vi "coincidenceVsDelay.vi"() -> ()   [LabVIEW 2020]
uses:
  <vilib>/Math Plots/2D Math Plots/2D Error Bar/2D Error Bar XCtrl/2D Error Bar.xctl
  C:/Program Files/Dotfast Consulting/Timetag Explorer 2.26/ttInterface.dll
  Program Files/Dotfast Consulting/Timetag Explorer 2.26/ttInterface.dll
  <vilib>/Utility/file.llb/Write Delimited Spreadsheet (I64).vi
  <vilib>/Math Plots/2D Math Plots/2D Error Bar/2D Error Bar Datatype/Public/Plot Helper (Fixed).vi
  <vilib>/Analysis/NI_AALBase.lvlib
  <vilib>/Math Plots/2D Math Plots/2D Error Bar/2D Error Bar Datatype/2D Error Bar Datatype.lvclass
panel:
  in  "stop":bool
  in  "Boolean":bool=TRUE
  in  "Step Delay(ns)":dbl
  in  "Stop Delay (ns)":dbl
  in  "StartDelay (ns)":dbl
  in  "fileName":string
  in  "Folder":path
  out "ChB Delay (uqd Unit)":i32
  out "ChADelay(uqd Unit)":i32
  in  "chB delay (ns)":dbl
  in  "chA delay(ns)":dbl
  in  "Ch B":u8=1 min=1 max=16 step=1
  in  "Ch A":u8=1 min=1 max=16 step=1
  out "CTW (uqd units)":i32
  in  "CTW in ns":dbl
  out "2D Error Bar":refnum<class "2D Plot Datatype.lvclass">[](xcontrol)
  out "Coincidence Rate AvsB":dbl format="%#_4p"
  out "ChB Rate":dbl format="%#_4p"
  out "ChARate":dbl format="%#_4p"
  out "Coincidence AvsB":i32
  out "Ch A":i32
  out "GetTimeCounter":i32
  out "Ch B":i32
  out "GetResolution":dbl
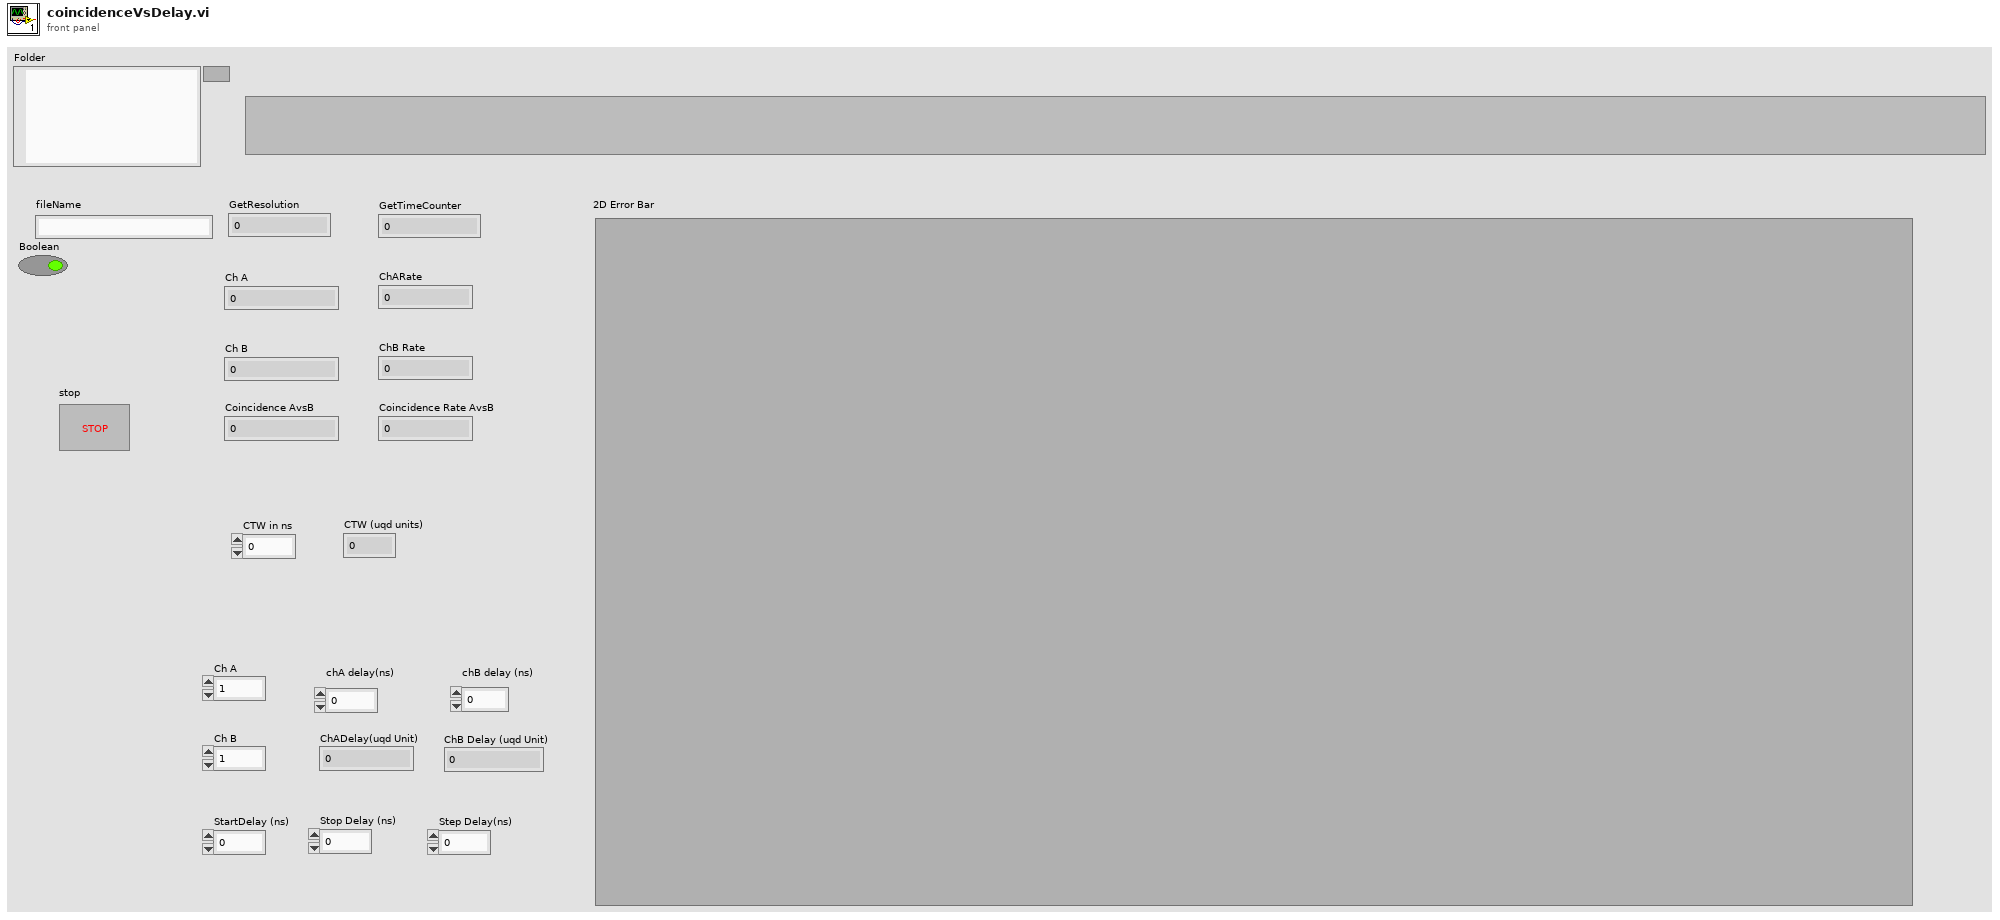
[diagram p1: front panel]
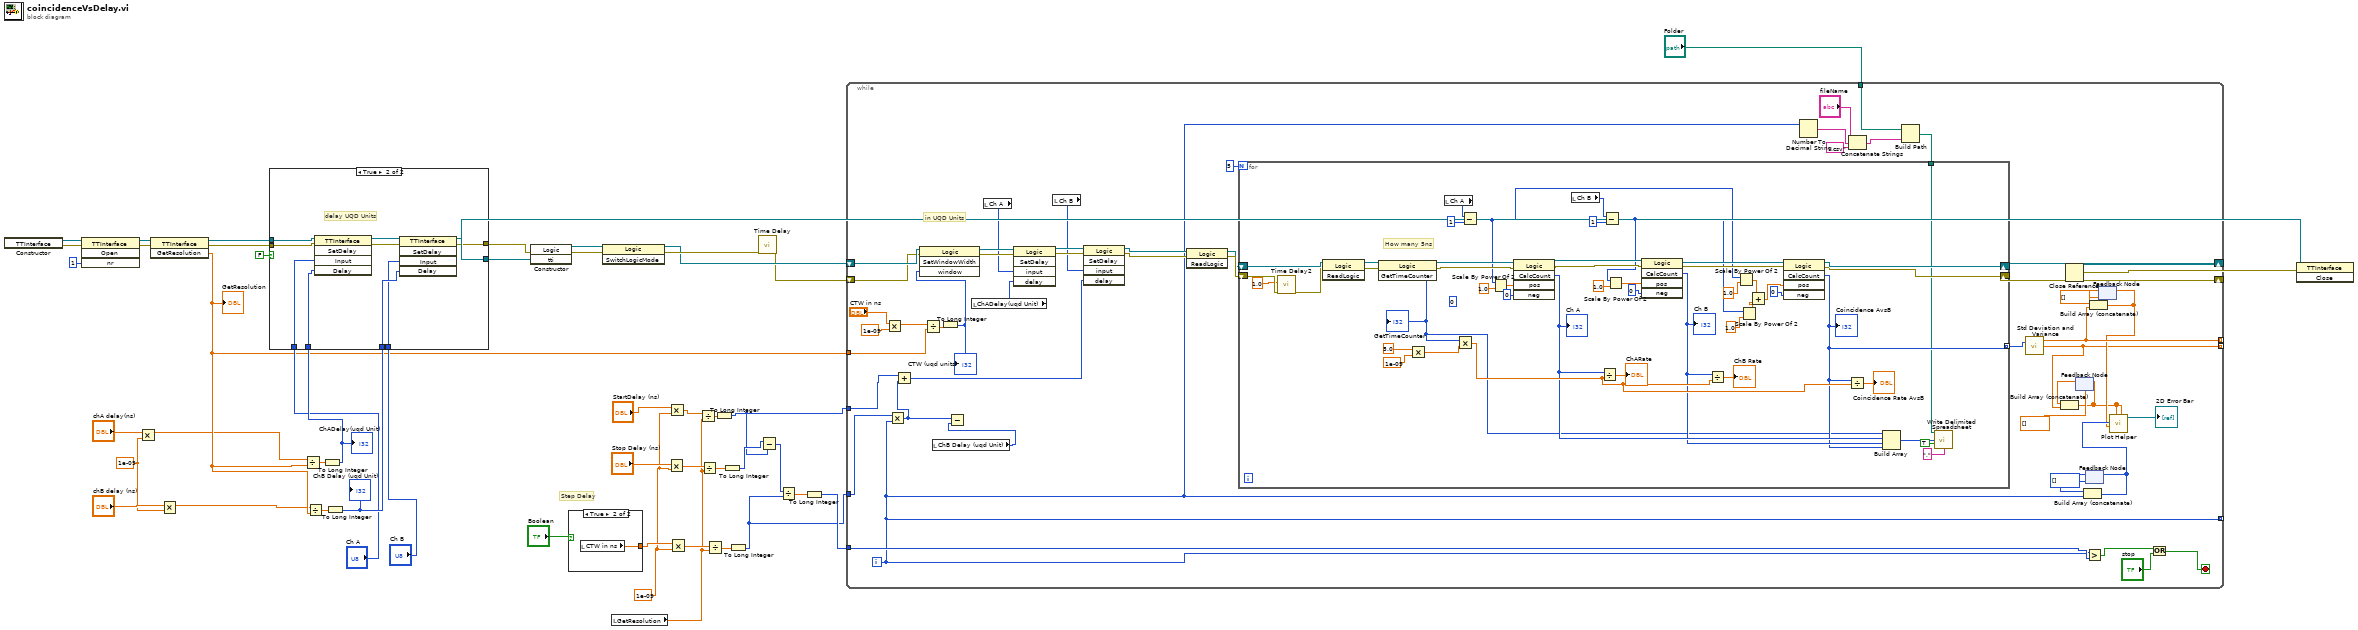
[diagram p0: block diagram]
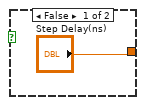
[diagram p2: hidden frame]
diagram:
  w14 = 1e-09
  w20 = 1e-09
  # "Step Delay"
  n1 = constructor class="TTInterface"() -> (reference out=w49:refnum<k24>, error out=w48:errorcluster)  [unwired: 3 in, 1 out]
  n2 = invoke class="TTInterface" method="Open"(reference=w49, error in=w48, "nr"=1) -> (reference out=w45:refnum<k24>, error out=w46:errorcluster)  [unwired: 1 in, 2 out]
  n3 = Multiply(x="chA delay(ns)", y=w20) -> (x*y=w22:dbl)
  n4 = invoke class="TTInterface" method="GetResolution"(reference=w45, error in=w46) -> (reference out=w44:refnum<k24>, error out=w43:errorcluster, "GetResolution"=w23:dbl)  [unwired: 1 in]
  "GetResolution" <- w23
  n5 = Multiply(x="chB delay (ns)", y=w20) -> (x*y=w21:dbl)
  n6 = Divide(x=w22, y=w23) -> (x/y=w29:dbl)
  n7 = Divide(x=w21, y=w23) -> (x/y=w28:dbl)
  n8 = To Long Integer(number=w29) -> (32bit integer=w27:i32)
  "ChADelay(uqd Unit)" <- w27
  n9 = To Long Integer(number=w28) -> (32bit integer=w26:i32)
  "ChB Delay (uqd Unit)" <- w26
  n10 = case shown="True" FALSE {
    tunnel: w44 -> [w51 w61]
    tunnel: w43 -> [w50 w60]
    tunnel: [w50 w57] -> w42
    tunnel: [w51 w56] -> w39
    tunnel: w27 -> [_ w55]
    tunnel: w26 -> [_ w54]
    tunnel: "Ch A" -> [_ w53]
    tunnel: "Ch B" -> [_ w52]
    frame False {
    }
    frame True {
      # "delay UQD Units"
      n11 = invoke class="TTInterface" method="SetDelay"(reference=w61, error in=w60, "Input"=w53, "Delay"=w55) -> (reference out=w59:refnum<k24>, error out=w58:errorcluster)  [unwired: 1 in, 3 out]
      n12 = invoke class="TTInterface" method="SetDelay"(reference=w59, error in=w58, "Input"=w52, "Delay"=w54) -> (reference out=w56:refnum<k24>, error out=w57:errorcluster)  [unwired: 1 in, 3 out]
    }
  }
  n13 = constructor class="Logic"(error in=w42, "tti"=w39) -> (reference out=w41:refnum<k24>, error out=w40:errorcluster)  [unwired: 2 in, 2 out]
  n14 = case shown="True" "Boolean" {
    tunnel: ["Step Delay(ns)" w63] -> w15
    frame False {
    }
    frame True {
      n15 = local read "CTW in ns"() -> (w63:dbl)
    }
  }
  n16 = invoke class="Logic" method="SwitchLogicMode"(reference=w41, error in=w40) -> (reference out=w34:refnum<k24>, error out=w35:errorcluster)  [unwired: 1 in, 1 out]
  n17 = local read "GetResolution"() -> (w10:dbl)
  n18 = Multiply(x="Stop Delay (ns)", y=w14) -> (x*y=w11:dbl)
  n19 = Multiply(x="StartDelay (ns)", y=w14) -> (x*y=w13:dbl)
  n20 = Multiply(x=w15, y=w14) -> (x*y=w12:dbl)
  n21 = Divide(x=w13, y=w10) -> (x/y=w9:dbl)
  n22 = Divide(x=w11, y=w10) -> (x/y=w8:dbl)
  n23 = Divide(x=w12, y=w10) -> (x/y=w7:dbl)
  n24 = To Long Integer(number=w9) -> (32bit integer=w3:i32)
  n25 = To Long Integer(number=w8) -> (32bit integer=w4:i32)
  n26 = To Long Integer(number=w7) -> (32bit integer=w1:i32)
  n27 = call "Time Delay"("error in (no error)"=w35) -> ("error out"=w33:errorcluster)  [unwired: 10 in]
  n28 = Subtract(x=w4, y=w3) -> (x-y=w6:i32)
  n29 = Divide(x=w6, y=w1) -> (x/y=w5:dbl)
  n30 = To Long Integer(number=w5) -> (32bit integer=w2:i32)
  n31 = while {
    shift-right: [w114] -> w37
    shift-left: w34 -> [w109]
    shift-right: [w113] -> w36
    shift-left: w33 -> [w108]
    tunnel: [w89] -> _ mode=indexing
    tunnel: [w86] -> _ mode=indexing
    tunnel: [w67] -> _ mode=indexing
    tunnel: w23 -> [w98]
    tunnel: "Folder" -> [w80]
    tunnel: w3 -> [w66]
    tunnel: w2 -> [w71]
    tunnel: w1 -> [w68]
    i -> [w67]
    stop <- w73 stop-if-true
    # "in UQD Units"
    n32 = Multiply(x="CTW in ns", y=1e-09) -> (x*y=w97:dbl)
    n33 = Multiply(x=w68, y=w67) -> (x*y=w65:i32)
    n34 = Add(x=w66, y=w65) -> (x+y=w64:i32)
    n35 = Divide(x=w97, y=w98) -> (x/y=w99:dbl)
    n36 = local read "ChB Delay (uqd Unit)"() -> (w74:i32)
    n37 = To Long Integer(number=w99) -> (32bit integer=w95:i32)
    "CTW (uqd units)" <- w95
    n38 = invoke class="Logic" method="SetWindowWidth"(reference=w109, error in=w108, "window"=w95) -> (reference out=w107:refnum<k24>, error out=w106:errorcluster)  [unwired: 1 in, 2 out]
    n39 = Subtract(x=w65, y=w74) -> ()  [unwired: 1 out]
    n40 = local read "ChADelay(uqd Unit)"() -> (w69:i32)
    n41 = local read "Ch A"() -> (w82:u8)
    n42 = invoke class="Logic" method="SetDelay"(reference=w107, error in=w106, "input"=w82, "delay"=w69) -> (reference out=w103:refnum<k24>, error out=w102:errorcluster)  [unwired: 1 in, 3 out]
    n43 = local read "Ch B"() -> (w81:u8)
    n44 = invoke class="Logic" method="SetDelay"(reference=w103, error in=w102, "input"=w81, "delay"=w64) -> (reference out=w105:refnum<k24>, error out=w104:errorcluster)  [unwired: 1 in, 3 out]
    n45 = invoke class="Logic" method="ReadLogic"(reference=w105, error in=w104) -> (reference out=w111:refnum<k24>, error out=w112:errorcluster)  [unwired: 1 in, 1 out]
    n46 = Number To Decimal String(number=w67) -> (decimal integer string=w77:string)  [unwired: 1 in]
    n47 = Concatenate Strings("fileName", w77, ".csv" ("string")) -> (w78:string)
    n48 = Build Path(base path=w80, name or relative path=w78) -> (appended path=w79:path)
    n49 = for {
      N: 5 -> [_]
      shift-right: [w138] -> w113
      shift-left: w112 -> [w158]
      shift-right: [w139] -> w114
      shift-left: w111 -> [w157]
      tunnel: [w120] -> w101 mode=indexing
      tunnel: w79 -> [w115]
      (unwired) u8 0 ("y")
      # "How many 5ns"
      n50 = call "Time Delay2"("error in (no error)"=w158, "Delay Time (s)"=1.0) -> ("error out"=w156:errorcluster)  [unwired: 9 in]
      n51 = invoke class="Logic" method="ReadLogic"(reference=w157, error in=w156) -> (reference out=w151:refnum<k24>, error out=w150:errorcluster)  [unwired: 1 in, 1 out]
      n52 = invoke class="Logic" method="GetTimeCounter"(reference=w151, error in=w150) -> (reference out=w146:refnum<k24>, error out=w145:errorcluster, "GetTimeCounter"=w118:i32)  [unwired: 1 in]
      "GetTimeCounter" <- w118
      n53 = Multiply(x=5.0, y=1e-09) -> (x*y=w152:dbl)
      n54 = local read "Ch A"() -> (w129:u8)
      n55 = Multiply(x=w118, y=w152) -> (x*y=w123:dbl)
      n56 = Subtract(x=w129, y=u8 1) -> (x-y=w125:u8)
      n57 = Scale By Power Of 2(n=w125, x=1.0) -> (x*2^n=w148:dbl)
      n58 = invoke class="Logic" method="CalcCount"(reference=w146, error in=w145, "pos"=w148, "neg"=0) -> (reference out=w144:refnum<k24>, error out=w143:errorcluster, "CalcCount"=w122:i32)  [unwired: 1 in, 2 out]
      "Ch A" <- w122
      n59 = local read "Ch B"() -> (w127:u8)
      n60 = Divide(x=w122, y=w123) -> (x/y=→"ChARate":dbl)
      n61 = Subtract(x=w127, y=u8 1) -> (x-y=w124:u8)
      n62 = Scale By Power Of 2(n=w124, x=1.0) -> (x*2^n=w160:dbl)
      n63 = invoke class="Logic" method="CalcCount"(reference=w144, error in=w143, "pos"=w160, "neg"=0) -> (reference out=w141:refnum<k24>, error out=w140:errorcluster, "CalcCount"=w121:i32)  [unwired: 1 in, 2 out]
      "Ch B" <- w121
      n64 = Divide(x=w121, y=w123) -> (x/y=→"ChB Rate":dbl)
      n65 = Scale By Power Of 2(n=w125, x=1.0) -> (x*2^n=w135:dbl)
      n66 = Scale By Power Of 2(n=w124, x=1.0) -> (x*2^n=w134:dbl)
      n67 = Add(x=w135, y=w134) -> (x+y=w133:dbl)
      n68 = invoke class="Logic" method="CalcCount"(reference=w141, error in=w140, "pos"=w133, "neg"=0) -> (reference out=w139:refnum<k24>, error out=w138:errorcluster, "CalcCount"=w120:i32)  [unwired: 1 in, 2 out]
      "Coincidence AvsB" <- w120
      n69 = Divide(x=w120, y=w123) -> (x/y=→"Coincidence Rate AvsB":dbl)
      n70 = Build Array(w118, w122, w121, w120) -> (w119:i32[])
      n71 = call-poly <vilib>:"Write Delimited Spreadsheet.vi"("file path (dialog if empty)"=w115, "1D data"=w119, "append to file? (new file:F)"=TRUE, "delimiter (\\t)"="," ("delimiter (\\t)")) -> ()  [unwired: 10 in, 2 out]
    }
    n72 = call <vilib>:"Std Deviation and Variance.vi"("X"=w101) -> ("mean"=w89:dbl, "standard deviation"=w86:dbl)  [unwired: 1 in, 1 out]
    n73 = feedback #1(dbl[] []) -> (w85:dbl[])
    n74 = Build Array (concatenate)(w85, w86) -> (w83:dbl[])
    n75 = feedback-in #1(w83) -> ()
    n76 = feedback #2(i32[] []) -> (w93:i32[])
    n77 = Build Array (concatenate)(w93, w67) -> (w91:i32[])
    n78 = feedback-in #2(w91) -> ()
    n79 = Greater?(x=w67, y=w71) -> (0:w70:bool)
    n80 = feedback #3(dbl[] []) -> (w90:dbl[])
    n81 = Build Array (concatenate)(w90, w89) -> (w88:dbl[])
    n82 = feedback-in #3(w88) -> ()
    n83 = call-poly <vilib>:"Plot Helper.vi"("error b vector"=w83, "error a vector"=w83, "y vector"=w88, "x vector"=w91) -> ("2D Plot Class Obj Array out"=→"2D Error Bar":refnum<class "2D Plot Datatype.lvclass">[])  [unwired: 2 in, 5 out]
    n84 = Or(x=w70, y="stop") -> (x .or. y?=w73:bool)
  }
  n85 = Close Reference(reference=w37, error in (no error)=w36) -> (error out=w38:errorcluster)
  n86 = invoke class="TTInterface" method="Close"(reference=w39, error in=w38) -> ()  [unwired: 1 in, 3 out]
